vi "refresh table.vi"(7 "Filter":string, 8 "error in":errorcluster, 9 "Table":refnum<vi>, 10 "taglist":refnum<data-value>, 11 "engine configuration in":refnum<class "engine configuration.lvclass">) -> (0 "error out":errorcluster)   [LabVIEW 2013, in "PL Framework Configuration Tool.lvlib" / "EngineTags.lvclass"]
uses:
  EngineTags.lvclass
  <vilib>/NI/Module Execution Interface/Engine Configuration/engine configuration.lvclass
  <vilib>/NI/Module Execution Interface/Engine Configuration/engine configuration.lvclass/engine configuration.ctl
  <vilib>/NI/Tag Bus/tag/tag descriptor.lvclass/tag descriptor.ctl
  EngineTags.lvclass/EngineTags.ctl
  <vilib>/NI/Tag Bus/tag/read tag name.vi
  <vilib>/NI/Tag Bus/tag/read data type.vi
  <vilib>/NI/Tag Bus/tag/read metadata.vi
  Read Sorting Enabled.vi
  Read Sorting Column.vi
  <vilib>/NI/Tag Bus/tag/tag descriptor.lvclass
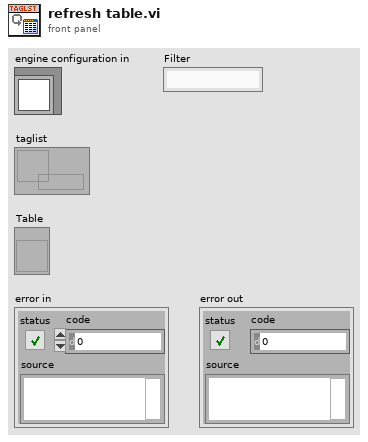
[diagram p1: front panel]
types:
  T1 = typedef "tag bus.lvlib/tag descriptor.lvclass/Data Type.ctl" = enum16{"Double", "Single", "I64", "I32", "I16", "I8", "U64", "U32", "U16", "U8", "Boolean", "String", "Array of Double", "Array of Single", "Array of I64", "Array of I32", "Array of I16", "Array of I8", "Array of U64", "Array of U32", "Array of U16", "Array of U8", "Array of Boolean", "Array of String"}
  T2 = typedef "sorting type.ctl" = enum16{"none", "asc", "desc"}
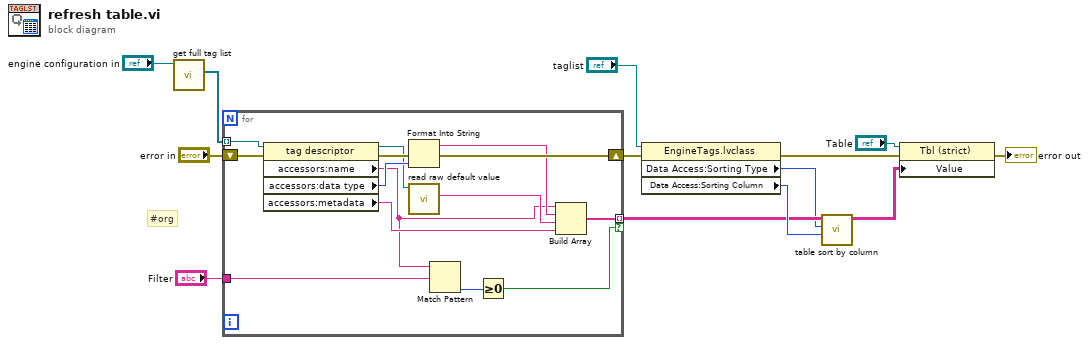
[diagram p0: block diagram]
diagram:
  # "#org"
  n1 = call <vilib>:"get full tag list.vi"("engine configuration in"="engine configuration in") -> ("tag list"=w6:refnum<class "tag descriptor.lvclass">[])  [unwired: 9 in, 1 out]
  n2 = for {
    shift-right: [w24] -> w4
    shift-left: "error in" -> [w27]
    tunnel: w6 -> [w26] mode=indexing
    tunnel: [w18] -> w8 mode=indexing if=w16
    tunnel: "Filter" -> [w14]
    n3 = property class="tag descriptor"(reference=w26, error in=w27) -> (reference out=w22:refnum<class "tag descriptor.lvclass">, error out=w25:errorcluster, "accessors:name"=w15:string, "accessors:data type"=w23:T1, "accessors:metadata"=w20:string)
    n4 = Format Into String(error in=w25, w23) -> (resulting string=w21:string, error out=w24:errorcluster)  [unwired: 2 in]
    n5 = call <vilib>:"read raw default value.vi"("system tag in"=w22) -> ("raw default"=w19:string)  [unwired: 8 in, 2 out]
    n6 = Match Pattern(string=w15, regular expression=w14) -> (offset past match=w17:i32)  [unwired: 1 in, 3 out]
    n7 = Greater Or Equal To 0?(x=w17) -> (x >= 0?=w16:bool)
    n8 = Build Array(w15, w21, w19, w20) -> (w18:string[])
  }
  n9 = property class="EngineTags.lvclass"(reference="taglist", error in=w4) -> (error out=w3:errorcluster, "Data Access:Sorting Type"=w2:T2, "Data Access:Sorting Column"=w10:i32)  [unwired: 1 out]
  n10 = call "table sort by column.vi"("Column to sort"=w10, "Sorting Type"=w2, "Array"=w8) -> ("sorted array"=w13:string[][])  [unwired: 8 in]
  n11 = property on="Property Node" class="Tbl (strict)"(reference="Table", error in=w3, "Value"=w13) -> (error out=→"error out":errorcluster)  [unwired: 1 out]
